vi "JV analyzer.vi"() -> ()   [LabVIEW 2017]
uses:
  <vilib>/Utility/file.llb/Read Delimited Spreadsheet (string).vi
  <vilib>/Utility/file.llb/Write Delimited Spreadsheet (string).vi
panel:
  out "Total files":i32
  in  "Stop Button":bool
  in  "Click to start":bool
  in  "Output name":string="JV_summary"
  out "PCE":string[](array[string])
  out "FF":string[](array[string])
  out "JSC":string[](array[string])
  out "VOC":string[](array[string])
  in  "Drag a folder below":path
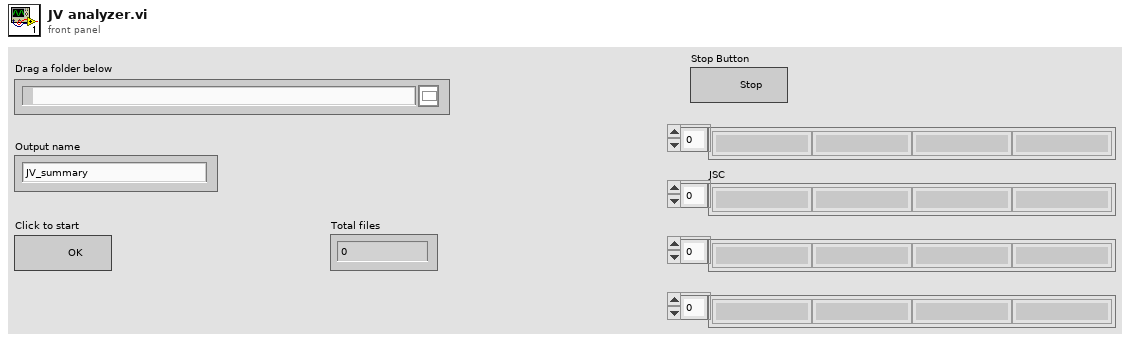
[diagram p1: front panel]
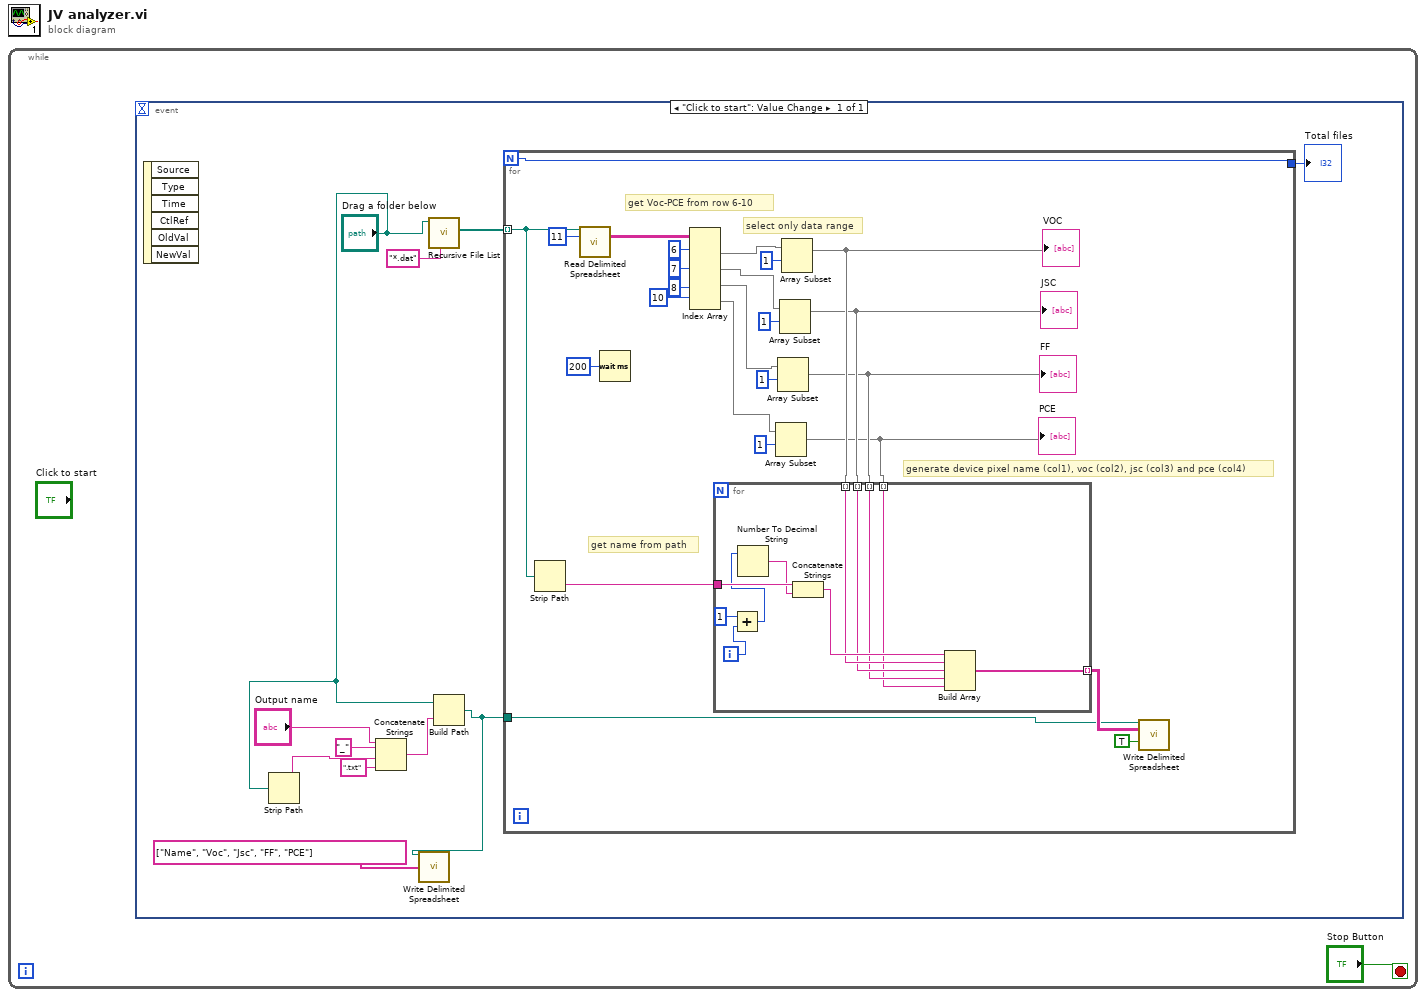
[diagram p0: block diagram]
diagram:
  n1 = while {
    stop <- "Stop Button" stop-if-true
    n2 = event shown="[0] \"Click to start\": Value Change" {
      selector: _ -> [_]
      dyn-events: _ -> [_]
      timeout: _ -> [_]
      event "Click to start": Value Change {
        n3 = event-data() -> ()  [unwired: 1 in, 6 out]
        n4 = Strip Path(path="Drag a folder below") -> (name=w10:string)  [unwired: 1 out]
        n5 = Concatenate Strings("Output name", "_" ("string"), w10, ".txt" ("string")) -> (w9:string)
        n6 = call <vilib>:"Recursive File List.vi"("pattern"="*.dat", "Folder Path"="Drag a folder below") -> ("All Files in Dir"=w11:path[])  [unwired: 5 in, 4 out]
        n7 = Build Path(base path="Drag a folder below", name or relative path=w9) -> (appended path=w5:path)
        n8 = call-poly <vilib>:"Write Delimited Spreadsheet.vi"("file path (dialog if empty)"=w5, "1D data"=string[] ["Name", "Voc", "Jsc", "FF", "PCE"] ("Header")) -> ()  [unwired: 12 in, 2 out]
        n9 = for {
          N -> [w13]
          tunnel: w11 -> [w17] mode=indexing
          tunnel: w5 -> [w14]
          tunnel: [w13] -> w2
          # "generate device pixel name (col1), voc (col2), jsc (col3) and pce (col4)"
          # "select only data range"
          # "get Voc-PCE from row 6-10"
          # "get name from path"
          n10 = Strip Path(path=w17) -> (name=w18:string)  [unwired: 1 out]
          n11 = call-poly <vilib>:"Read Delimited Spreadsheet.vi"("file path (dialog if empty)"=w17, "number of rows (all:-1)"=11) -> ("all rows"=w35:string[][])  [unwired: 8 in, 5 out]
          n12 = Wait (ms)(milliseconds to wait=u32 200) -> ()  [unwired: 1 out]
          n13 = Index Array(array=w35, index (row) #1=6 ("index (row)"), index (row) #2=7 ("index (row)"), index (row) #3=8 ("index (row)"), index (row) #4=10 ("index (row)")) -> (element #1=w26:string[], element #2=w25:string[], element #3=w24:string[], element #4=w23:string[])  [unwired: 4 in]
          n14 = Array Subset(array=w23, index=1) -> (w19:string[])  [unwired: 1 in]
          "PCE" <- w19
          n15 = Array Subset(array=w24, index=1) -> (w20:string[])  [unwired: 1 in]
          "FF" <- w20
          n16 = Array Subset(array=w25, index=1) -> (w21:string[])  [unwired: 1 in]
          "JSC" <- w21
          n17 = Array Subset(array=w26, index=1) -> (w22:string[])  [unwired: 1 in]
          "VOC" <- w22
          n18 = for {
            tunnel: w22 -> [w42] mode=indexing
            tunnel: w21 -> [w41] mode=indexing
            tunnel: w20 -> [w40] mode=indexing
            tunnel: w19 -> [w39] mode=indexing
            tunnel: w18 -> [w48]
            tunnel: [w38] -> w15 mode=indexing
            i -> [w46]
            n19 = Add(x=1, y=w46) -> (x+y=w44:i32)
            n20 = Number To Decimal String(number=w44) -> (decimal integer string=w47:string)  [unwired: 1 in]
            n21 = Concatenate Strings(w48, w47) -> (w43:string)
            n22 = Build Array(w43, w42, w41, w40, w39) -> (w38:string[])
          }
          n23 = call-poly <vilib>:"Write Delimited Spreadsheet.vi"("file path (dialog if empty)"=w14, "2D data"=w15, "append to file? (new file:F)"=TRUE) -> ()  [unwired: 11 in, 2 out]
        }
        "Total files" <- w2
      }
    }
  }
